vi "5T_check_queue.vi"(7 "error in (no error)":errorcluster, 10 "Queue":refnum<queue> caption="5T Queue") -> (0 "error out":errorcluster, 1 "5T Control":T1 {"Rate (T/min)" format="%6_5f"}, 3 "New Entries?":bool)   [LabVIEW 2019]
uses:
  Mischer/5T_Control.ctl
panel:
  out "Numeric":i32
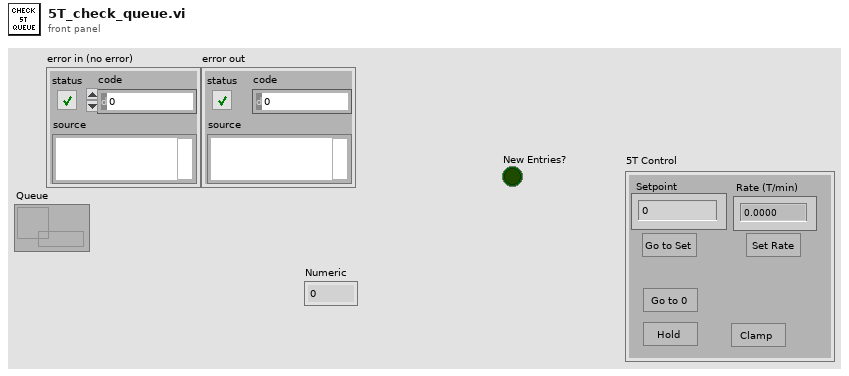
[diagram p1: front panel]
types:
  T1 = typedef "5T_Control.ctl" = cluster{"Rate (T/min)":dbl, "Setpoint":dbl, "Go to set":bool, "Go to Zero":bool, "Clamp":bool, "Go to Hold":bool, "Set Rate":bool}
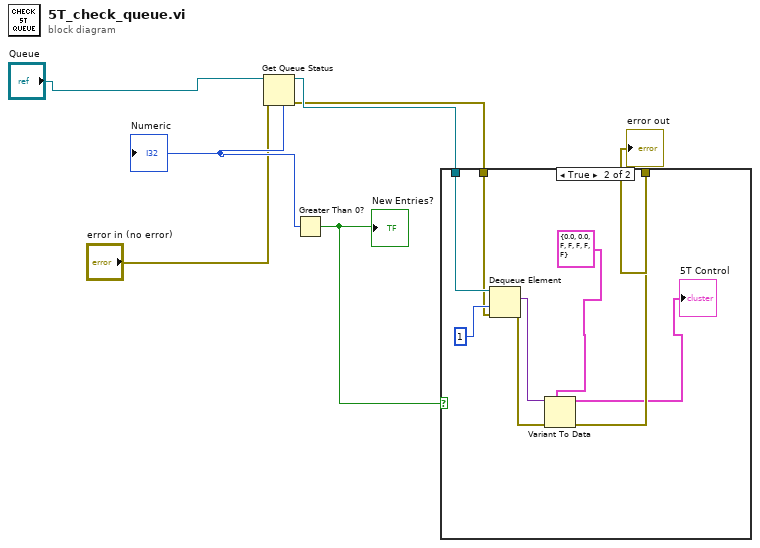
[diagram p0: block diagram]
diagram:
  n1 = Get Queue Status(queue="Queue", error in (no error)="error in (no error)") -> (queue out=w6:refnum<queue>, error out=w4:errorcluster, # elements in queue=w7:i32)  [unwired: 1 in, 5 out]
  "Numeric" <- w7
  n2 = Greater Than 0?(x=w7) -> (x > 0?=w5:bool)
  "New Entries?" <- w5
  n3 = case shown="True" w5 {
    tunnel: w6 -> [_ w14]
    tunnel: w4 -> [w8 w13]
    tunnel: [w8 w11] -> w2
    frame False {
    }
    frame True {
      n4 = Dequeue Element(queue=w14, timeout in ms (-1)=1, error in (no error)=w13) -> (element=w15:variant, error out=w12:errorcluster)  [unwired: 2 out]
      n5 = Variant To Data(error in=w12, type=T1 {"Rate (T/min)"=0.0, "Setpoint"=0.0, "Go to set"=FALSE, "Go to Zero"=FALSE, "Clamp"=FALSE, "Go to Hold"=FALSE, "Set Rate"=FALSE} ("5T Control 2"), Variant=w15) -> (data=→"5T Control":T1, error out=w11:errorcluster)
    }
  }
  "error out" <- w2
